vi "Normalize Const.vi"() -> (0 "Const":i32=1024)   [LabVIEW 2017, in "Measurement.PhotocurrentMapping.UI.lvclass"]
uses:
  Measurement.PhotocurrentMapping.UI.lvclass
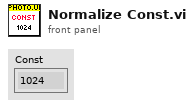
[diagram p1: front panel]
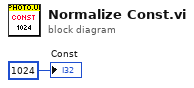
[diagram p0: block diagram]
diagram:
  "Const" <- 1024
